vi "Read_txt.vi"(0 "file path (dialog if empty)":path) -> (1 "Elements":string[][](array[string]), 2 "Rows":i32, 3 "Cols":i32)   [LabVIEW 2014]
uses:
  <vilib>/Utility/file.llb/Read From Spreadsheet File (string).vi
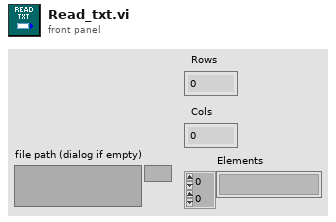
[diagram p1: front panel]
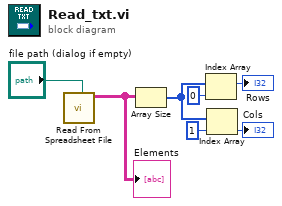
[diagram p0: block diagram]
diagram:
  n1 = call-poly <vilib>:"Read From Spreadsheet File.vi"("file path (dialog if empty)"="file path (dialog if empty)") -> ("all rows"=w3:string[][])  [unwired: 6 in, 4 out]
  "Elements" <- w3
  n2 = Array Size(array=w3) -> (size(s)=w5:i32[])
  n3 = Index Array(array=w5, index=0) -> (element=→"Rows":i32)
  n4 = Index Array(array=w5, index=1) -> (element=→"Cols":i32)
